vi "LoadRecentPrograms.vi"(0 "Program Interface in":refnum<class "Program Interface.lvclass">, 5 "error in (no error)":errorcluster) -> (14 "Program Interface out":refnum<class "Program Interface.lvclass">, 19 "error out":errorcluster)   [LabVIEW 2016, in "Program Interface.lvclass"]
uses:
  Program Interface.lvclass
  C:/_Code/Development/UR LabVIEW Interface/Classes/Application Interface/Application Interface.lvclass
  Program Interface.lvclass/Program Interface.ctl
  Application/Application.lvclass
  <vilib>/Utility/config.llb/NI_LVConfig.lvlib
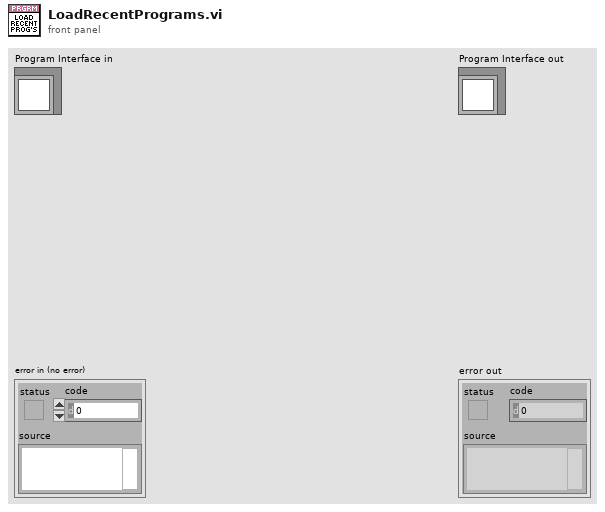
[diagram p1: front panel]
types:
  T1 = typedef "NI_LVConfig.lvlib/Config Data RefNum.ctl" = refnum<k1>
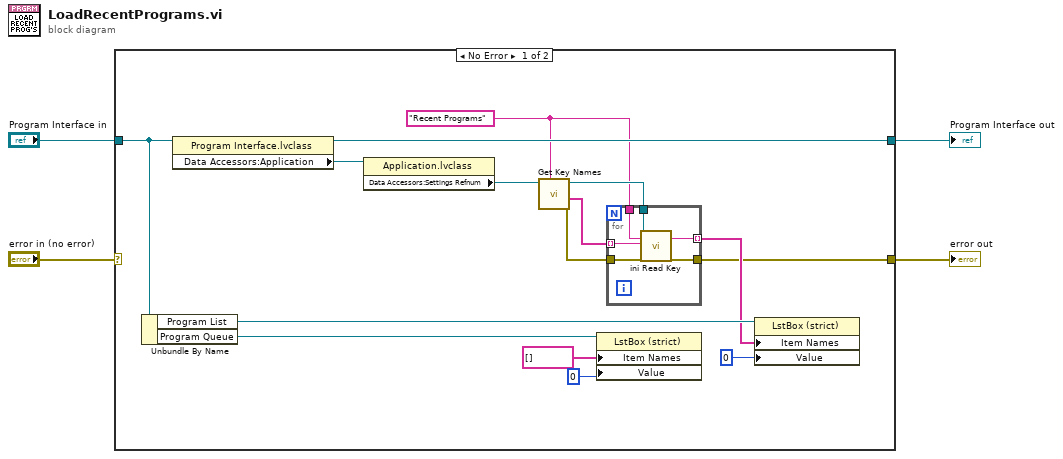
[diagram p0: block diagram]
diagram:
  n1 = case shown="No Error" "error in (no error)" {
    selector: "error in (no error)" -> [_ w27]
    tunnel: [w9 w27] -> w3
    tunnel: [w19 w26] -> w1
    tunnel: "Program Interface in" -> [w16 w26]
    frame No Error {
      w12 = "Recent Programs" ("section")
      n2 = Unbundle By Name(w16) -> ("Program List"=w11:refnum<vi>, "Program Queue"=w7:refnum<vi>)
      n3 = property class="Program Interface.lvclass"(reference=w16) -> (reference out=w19:refnum<class "Program Interface.lvclass">, "Data Accessors:Application"=w18:refnum<class "Application.lvclass">)  [unwired: 1 in, 1 out]
      n4 = property class="Application.lvclass"(reference=w18) -> ("Data Accessors:Settings Refnum"=w17:T1)  [unwired: 1 in, 2 out]
      n5 = call <vilib>:"Get Key Names.vi"("section"=w12, "refnum"=w17) -> ("error out"=w14:errorcluster, "key names"=w13:string[], "refnum out"=w15:T1)  [unwired: 6 in, 1 out]
      n6 = property class="LstBox (strict)"(reference=w7, "Item Names"=string[] [], "Value"=0) -> ()  [unwired: 1 in, 2 out]
      n7 = for {
        tunnel: w15 -> [w25]
        tunnel: w14 -> [w24]
        tunnel: w13 -> [w23] mode=indexing
        tunnel: w12 -> [w22]
        tunnel: [w21] -> w9
        tunnel: [w20] -> w10 mode=indexing
        n8 = call "ini Read Key.vi"("Refnum in"=w25, "Section"=w22, "Key"=w23, "Error In"=w24) -> ("value"=w20:string, "error out"=w21:errorcluster)  [unwired: 13 in, 1 out]
      }
      n9 = property class="LstBox (strict)"(reference=w11, "Item Names"=w10, "Value"=u16 0) -> ()  [unwired: 1 in, 2 out]
    }
    frame Error {
    }
  }
  "error out" <- w3
  "Program Interface out" <- w1
